vi "TB-Save Cal Signal.vi"(0 "Params":T1={"Low cutoff (kHz)"=0.0, "High cutoff (kHz)"=0.0, "Duration (min)"=0.0, "dB SPL"=100.0, "Waveform"=enum."Noise", "WAVfile"=path "", "refWav"=path "", "use mic correction"=FALSE, "micCorrFile"=path "", "Pistonphone Level (dB SPL)"=0.0, "Sampling rate (Hz)"=0.0, "Buffer length (s)"=0.0, "Stream mic"=FALSE, "Fine adjust"={"Max"=0.0, "Min"=0.0}, "Mic gain"=0.0, "atten"=0.0, "resol (Hz)"=0.0, "navgs"=0, "Allow Slack"=FALSE, "max starts"=0, "Freq (kHz)"=8.0, "Tma (s)"=0.0, "Streamed"=[], "Drive"=""}, 2 "ID":string, 9 "Mic signal":dbl[](array[numeric])) -> (15 "error out":errorcluster)   [LabVIEW 2020]
uses:
  Typedefs/TB-Parameters.ctl
  epl-vi-lib/Signal Synthesis VIs/Controls/Waveform XCtl/Waveform Enum.ctl
  <vilib>/sound2/lvsound2.llb/Sound Data Format.ctl
  <vilib>/sound2/lvsound2.llb/Sound File Write Open.vi
  <vilib>/sound2/lvsound2.llb/Sound File Write (DBL).vi
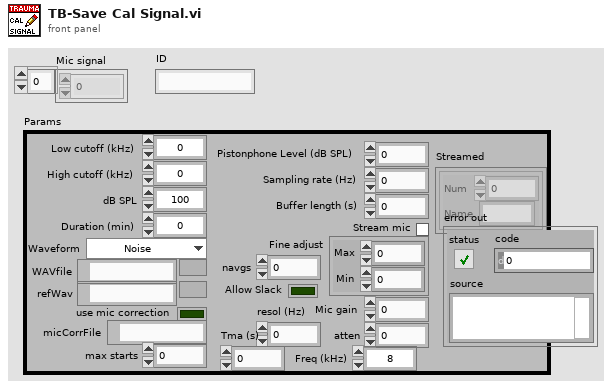
[diagram p1: front panel]
types:
  T1 = typedef "TB-Parameters.ctl" = cluster{"Low cutoff (kHz)":dbl, "High cutoff (kHz)":dbl, "Duration (min)":dbl, "dB SPL":dbl, "Waveform":T2, "WAVfile":path, "refWav":path, "use mic correction":bool, "micCorrFile":path, "Pistonphone Level (dB SPL)":dbl, "Sampling rate (Hz)":dbl, "Buffer length (s)":dbl, "Stream mic":bool, "Fine adjust":cluster{"Max":dbl, "Min":dbl}, "Mic gain":dbl, "atten":dbl, "resol (Hz)":dbl, "navgs":i32, "Allow Slack":bool, "max starts":i32, "Freq (kHz)":dbl, "Tma (s)":dbl, "Streamed":cluster{"Num":i32, "Name":string}[], "Drive":string}
  T2 = typedef "Waveform Enum.ctl" = enum16{"OFF", "Tone", "Noise", "Pulse Train", "File", "FM Sweep", "Chirp Train", "Complex Tone", "FM Tone", "Moving Ripple"}
  T3 = typedef "Sound Data Format.ctl" = cluster{"sample rate (S/s)":dbl, "number of channels":i32, "bits per sample":i32}
  T4 = typedef "Sound File Refnum.ctl" = refnum<file>
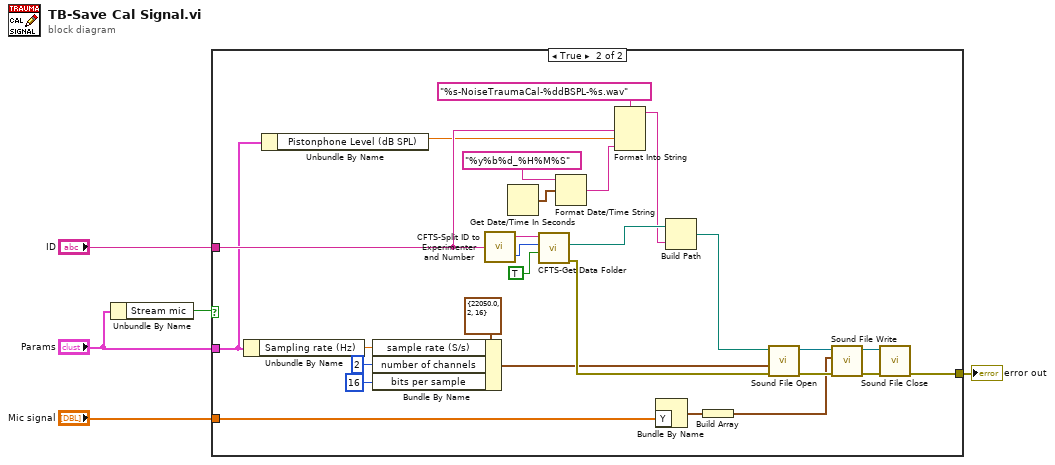
[diagram p0: block diagram]
diagram:
  n1 = Unbundle By Name("Params") -> ("Stream mic"=w5:bool)
  n2 = case shown="True" w5 {
    tunnel: "Params" -> [_ w8]
    tunnel: "ID" -> [_ w23]
    tunnel: "Mic signal" -> [_ w20]
    tunnel: [_ w6] -> w1
    frame False {
    }
    frame True {
      n3 = Unbundle By Name(w8) -> ("Sampling rate (Hz)"=w7:dbl)
      n4 = Unbundle By Name(w8) -> ("Pistonphone Level (dB SPL)"=w22:dbl)
      n5 = Bundle By Name(cluster=T3 {"sample rate (S/s)"=22050.0, "number of channels"=2, "bits per sample"=16} ("sound format"), "sample rate (S/s)"=w7, "number of channels"=2, "bits per sample"=16) -> (w11:T3)
      n6 = call "CFTS-Split ID to Experimenter and Number.vi"("ID"=w23) -> ("Experimenter"=w31:string, "Number"=w32:i32)
      n7 = Get Date/Time In Seconds() -> (seconds since 1Jan1904=w27:timestamp)
      n8 = call "CFTS-Get Data Folder.vi"("create?"=TRUE, "Number"=w32, "Experimenter"=w31) -> ("error out"=w14:errorcluster, "Data folder"=w30:path)  [unwired: 7 in]
      n9 = Format Date/Time String(time format string (%c)="%y%b%d_%H%M%S", seconds (now)=w27) -> (date/time string=w24:string)  [unwired: 1 in]
      n10 = Format Into String(format string="%s-NoiseTraumaCal-%ddBSPL-%s.wav", w23, w22, w24) -> (resulting string=w28:string)  [unwired: 2 in, 1 out]
      n11 = Bundle By Name("Y"=w20) -> (w21:waveform(dbl))  [unwired: 1 in]
      n12 = Build Path(base path=w30, name or relative path=w28) -> (appended path=w19:path)
      n13 = Build Array(w21) -> (w13:waveform(dbl)[])
      n14 = call-poly <vilib>:"Sound File Open.vi"("error in (no error)"=w14, "sound format"=w11, "path"=w19) -> ("error out"=w16:errorcluster, "sound file refnum"=w18:T4)  [unwired: 7 in]
      n15 = call-poly <vilib>:"Sound File Write.vi"("error in (no error)"=w16, "data"=w13, "sound file refnum"=w18) -> ("error out"=w15:errorcluster, "sound file refnum out"=w17:T4)  [unwired: 7 in]
      n16 = call <vilib>:"Sound File Close.vi"("error in (no error)"=w15, "sound file refnum"=w17) -> ("error out"=w6:errorcluster)  [unwired: 9 in]
    }
  }
  "error out" <- w1
